vi "secureCopy.vi"(8 "error in (no error)":errorcluster, 10 "Item For Copy Selection":T1, 11 "FileTransfer in":refnum<class "FileTransfer.lvclass">) -> (0 "error out":errorcluster, 3 "FileTransfer out":refnum<class "FileTransfer.lvclass">)   [LabVIEW 2016, in "FileTransfer.lvclass"]
uses:
  FileTransfer.lvclass
  Typedefs/Item For Copy Selection.ctl
  FileTransfer.lvclass/FileTransfer.ctl
panel:
  out "standard error":string
  out "standard output":string
  out "return code":i32
  out "concatenated string":string
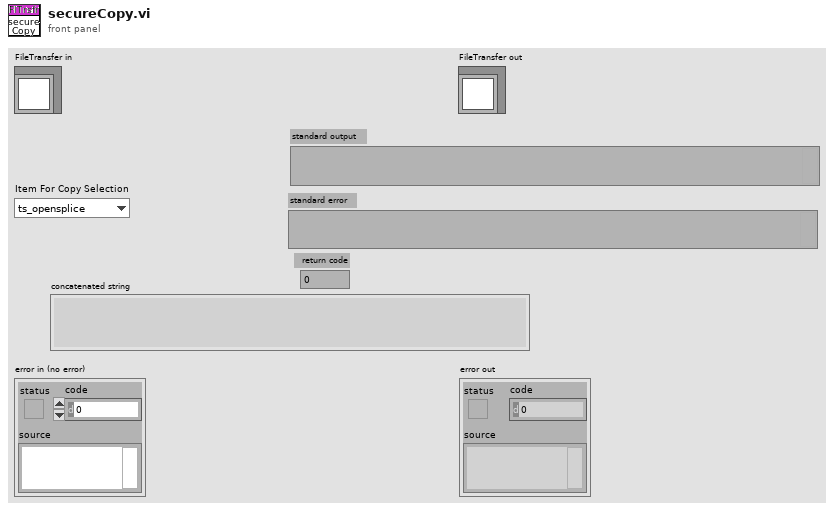
[diagram p1: front panel]
types:
  T1 = typedef "Item For Copy Selection.ctl" = enum16{"ts_opensplice", "ts_sal"}
  T2 = cluster{"Username":string, "IP Address":string, "Path to ts_opensplice source":path, "Path to ts_sal source":path}
  T3 = typedef "cRIO.ctl" = cluster{"Username":string, "IP Address":string, "Path to ts_opensplice target":path, "Path to ts_sal target":path}
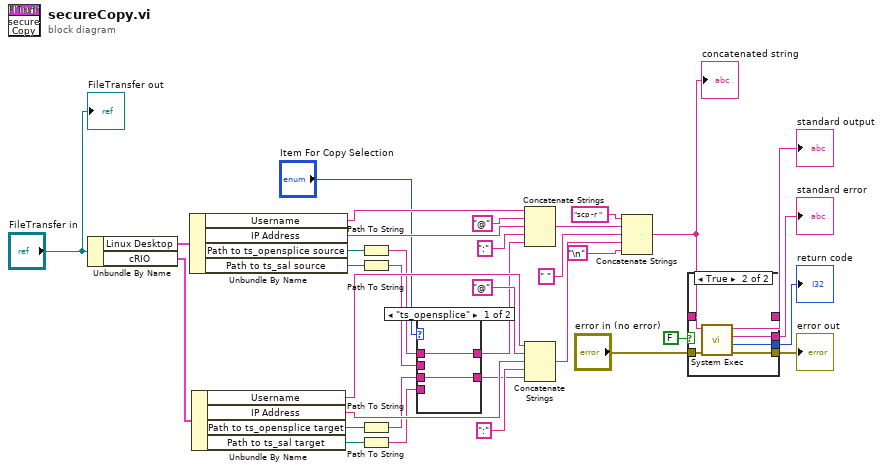
[diagram p0: block diagram]
diagram:
  n1 = Unbundle By Name("FileTransfer in") -> ("Linux Desktop"=w18:T2, "cRIO"=w17:T3)
  n2 = Unbundle By Name(w18) -> ("Username"=w33:string, "IP Address"=w32:string, "Path to ts_opensplice source"=w30:path, "Path to ts_sal source"=w15:path)
  n3 = Unbundle By Name(w17) -> ("Username"=w27:string, "IP Address"=w26:string, "Path to ts_opensplice target"=w28:path, "Path to ts_sal target"=w16:path)
  n4 = Path To String(path=w30) -> (string=w12:string)
  n5 = Path To String(path=w15) -> (string=w11:string)
  n6 = Path To String(path=w28) -> (string=w13:string)
  n7 = Path To String(path=w16) -> (string=w10:string)
  n8 = case shown="\"ts_opensplice\"" "Item For Copy Selection" {
    tunnel: w13 -> [w35 _]
    tunnel: w12 -> [w36 _]
    tunnel: w11 -> [_ w38]
    tunnel: w10 -> [_ w37]
    tunnel: [w36 w38] -> w9
    tunnel: [w35 w37] -> w8
    frame "ts_opensplice" {
    }
    frame "ts_sal" {
    }
  }
  n9 = Concatenate Strings(w33, "@" ("string"), w32, ":" ("string"), w9) -> (w22:string)
  n10 = Concatenate Strings(w27, "@" ("string"), w26, ":" ("string"), w8) -> (w20:string)
  n11 = Concatenate Strings("scp -r " ("string"), w22, " " ("string"), w20, "\n") -> (w7:string)
  "concatenated string" <- w7
  n12 = case shown="True" FALSE {
    tunnel: w7 -> [_ w45]
    tunnel: "error in (no error)" -> [w39 w44]
    tunnel: [w39 w43] -> w5
    tunnel: [_ w42] -> w4
    tunnel: [_ w41] -> w3
    tunnel: [_ w40] -> w2
    frame False {
    }
    frame True {
      n13 = call <vilib>:"System Exec.vi"("error in (no error)"=w44, "command line"=w45) -> ("error out"=w43:errorcluster, "return code"=w42:i32, "standard error"=w40:string, "standard output"=w41:string)  [unwired: 6 in]
    }
  }
  "error out" <- w5
  "return code" <- w4
  "standard output" <- w3
  "standard error" <- w2
  "FileTransfer out" <- "FileTransfer in"
